vi "Measurements UI_Measure-Scope SP.vi"() -> ()   [LabVIEW 2012]
uses:
  Measurement Operations_Meas.ctl
  Measure Operations_Meas.ctl
  Data Structure.llb/Sub Panel Status Flag_DStr-Scope SP.vi
  SCOPE Acquisition.llb/SCOPE Operations_SA-Scope SP.ctl
  <vilib>/Utility/miscctls.llb/LVStringsAndValuesArrayTypeDef.ctl
panel:
  in  "TempVari":T3={"error"={"status"=FALSE, "code"=0, "source"=""}, "Measure"=refnum, "Message"={"Chans"=[{"String"="0", "Value"=0.0}, {"String"="1", "Value"=1.0}], "LevelRange"={"Max"=10.0, "Min"=-10.0}, "InstruHandle"=""}, "message"=variant, "Item Names"=[], "Config"=[], "InstruHandle"=""}
  in  "Done":bool
  in  "Clear":bool
  in  "Remove":bool
  in  "Add":bool
  in  "List":i32(listbox) caption="标量测量"
  # "操作"
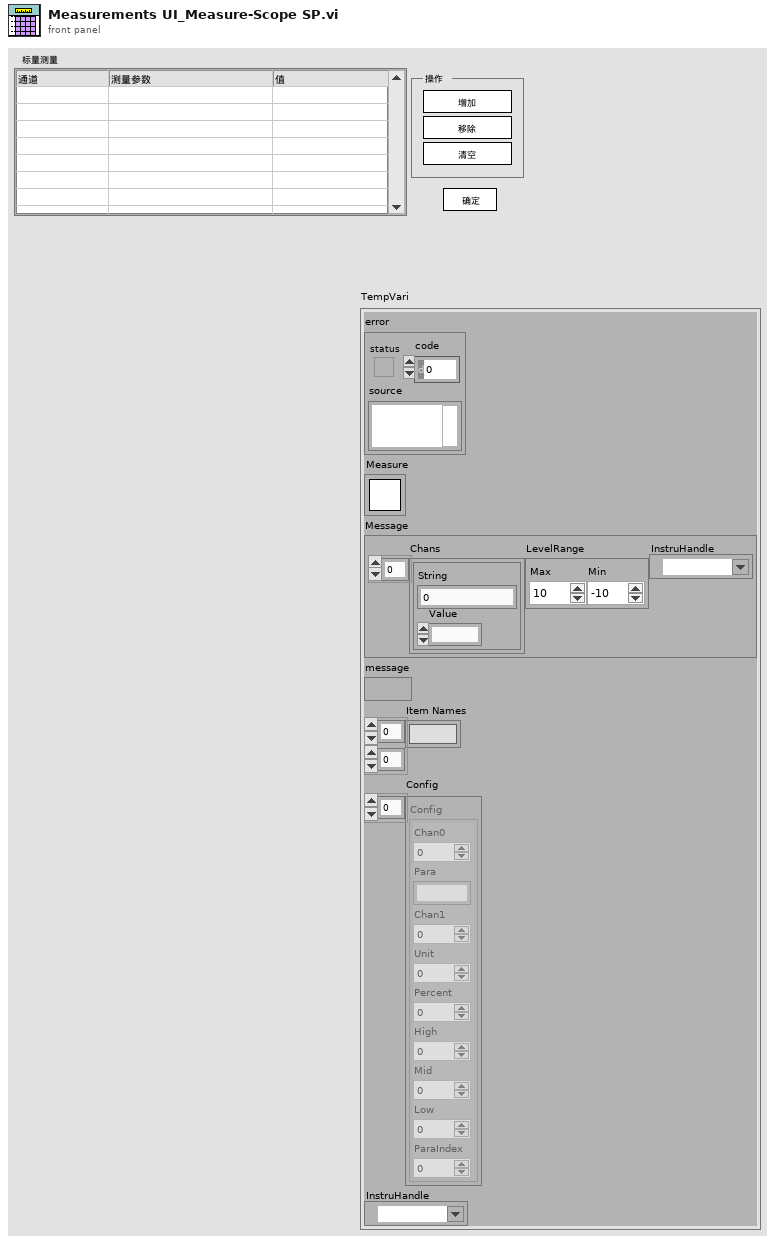
[diagram p1: front panel]
types:
  T1 = typedef "Queue RefNum" = refnum<k1>
  T2 = typedef "LVStringsAndValuesArrayTypeDef.ctl" = cluster{"String":string, "Value":ext}[]
  T3 = cluster{"error":errorcluster, "Measure":T1, "Message":cluster{"Chans":T2, "LevelRange":cluster{"Max":dbl, "Min":dbl}, "InstruHandle":refnum<k15>}, "message":variant, "Item Names":string[][], "Config":cluster{"Chan0":i32, "Para":string, "Chan1":i32, "Unit":i32, "Percent":i32, "High":dbl, "Mid":dbl, "Low":dbl, "ParaIndex":i32}[], "InstruHandle":refnum<k15>}
  T4 = typedef "Measurement Operations_Meas.ctl" = enum16{"Initialize", "Idle", "Add", "Delete", "Clear", "Caculate", "Refresh List Items", "Error Handle", "Close FP", "Exit"}
  T5 = typedef "Measure Operations_Meas.ctl" = enum16{"Add", "Config&Read", "Delete", "Clear"}
  T6 = typedef "SCOPE Operations_SA-Scope SP.ctl" = enum16{"Noop", "Initial", "Horizontal", "Vertical", "Trigger", "RIS", "Initiate", "Fetch", "Abort", "Close", "SelfCalibrate", "AutoSetup"}
  T7 = typedef "Dynamic VI Paths_FS-Scope SP.ctl" = cluster{"Measure":path, "Cursors":path, "Add Para":path, "Config":path}
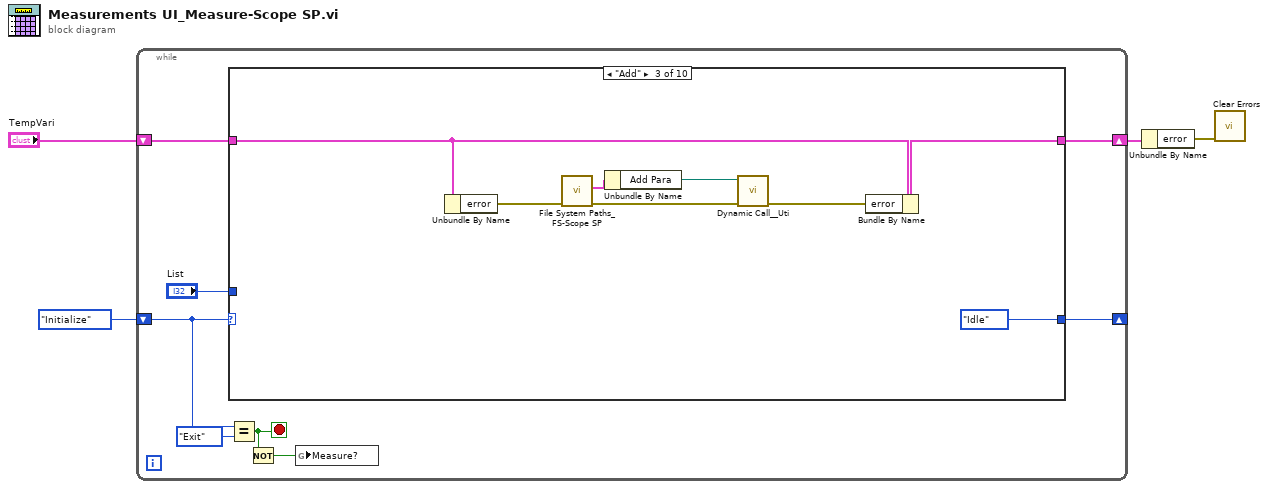
[diagram p0: block diagram]
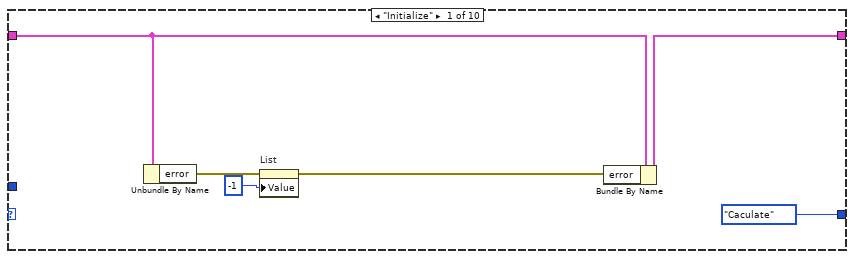
[diagram p2: hidden frame]
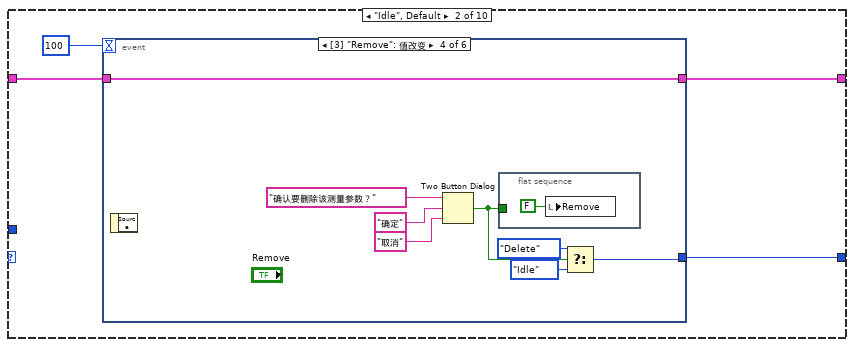
[diagram p3: hidden frame]
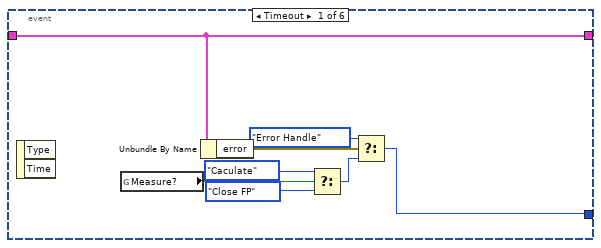
[diagram p4: hidden frame]
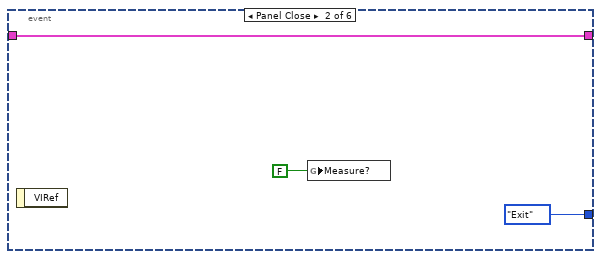
[diagram p5: hidden frame]
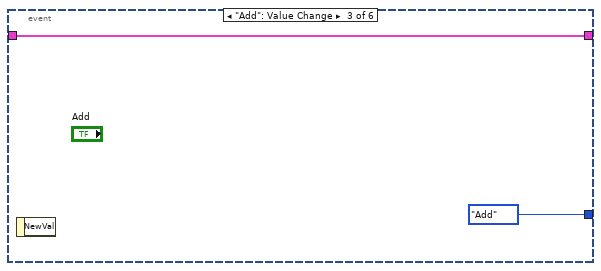
[diagram p6: hidden frame]
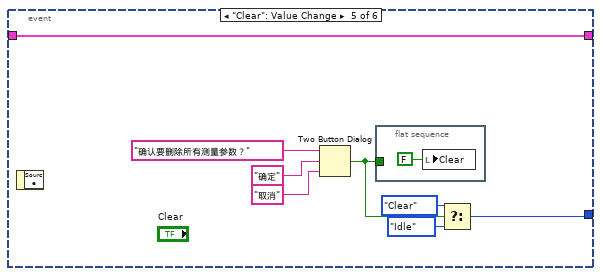
[diagram p7: hidden frame]
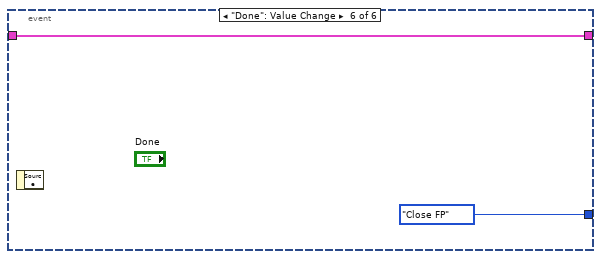
[diagram p8: hidden frame]
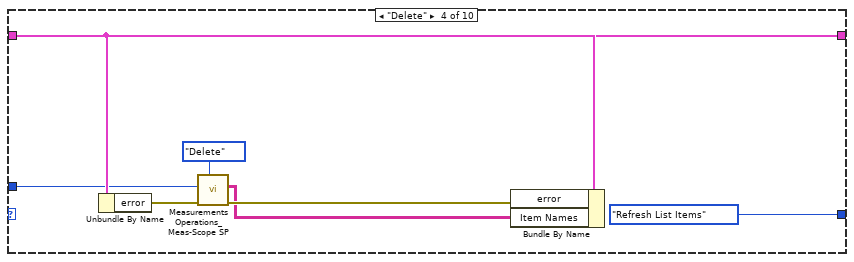
[diagram p9: hidden frame]
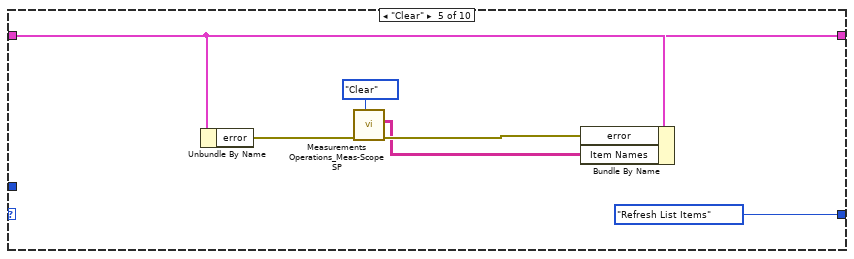
[diagram p10: hidden frame]
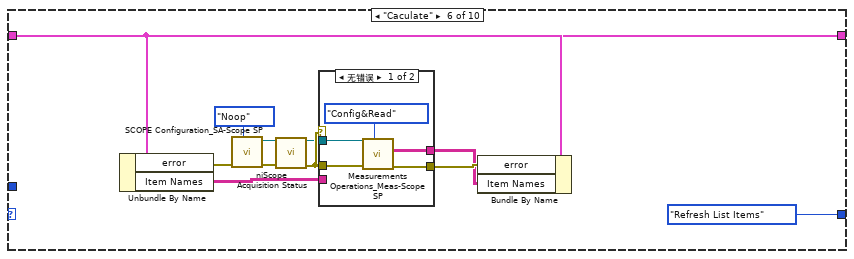
[diagram p11: hidden frame]
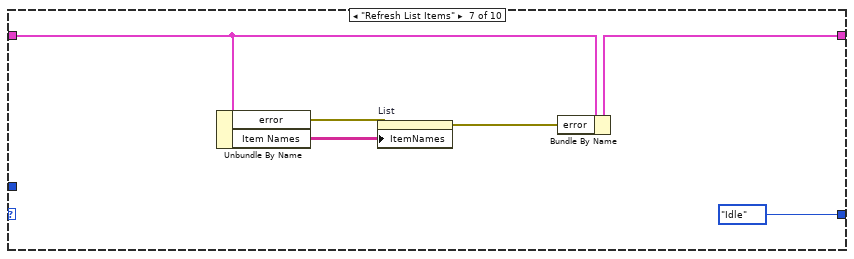
[diagram p13: hidden frame]
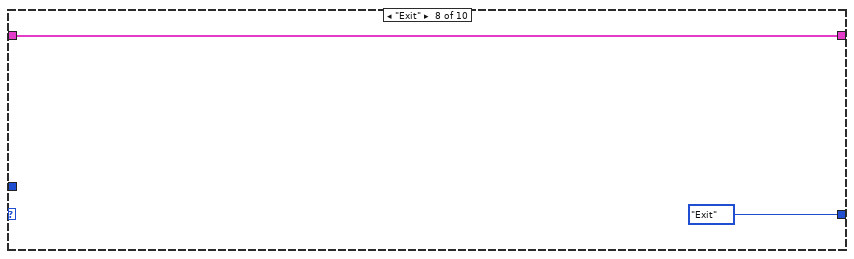
[diagram p14: hidden frame]
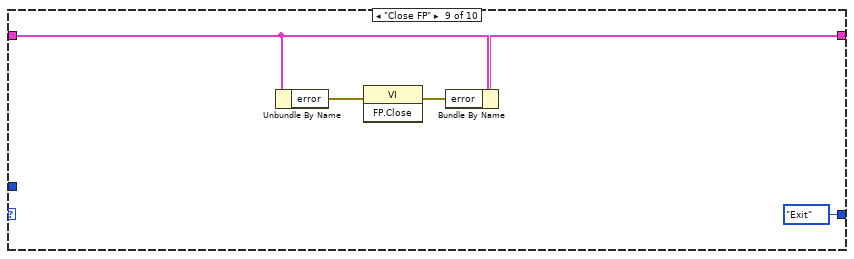
[diagram p15: hidden frame]
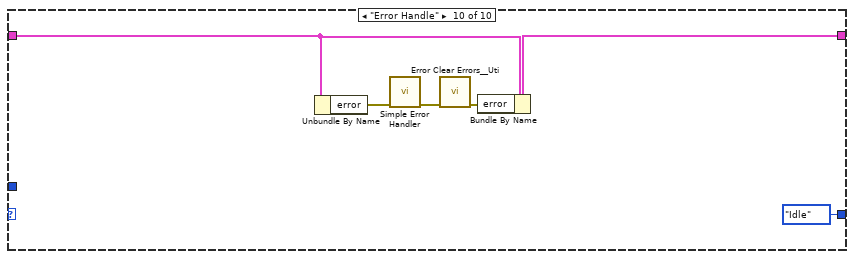
[diagram p16: hidden frame]
diagram:
  n1 = while {
    shift-right: [w12] -> _
    shift-left: Measurement_Operations_Meas."Initialize" ("Operations") -> [w11]
    shift-right: [w7] -> w3
    shift-left: "TempVari" -> [w8]
    stop <- w6 stop-if-true
    n2 = case shown="\"Add\"" w11 {
      tunnel: [Measurement_Operations_Meas."Caculate" ("Operations") w21 Measurement_Operations_Meas."Idle" ("Operations") Measurement_Operations_Meas."Refresh List Items" ("Operations") Measurement_Operations_Meas."Refresh List Items" ("Operations") Measurement_Operations_Meas."Refresh List Items" ("Operations") Measurement_Operations_Meas."Idle" ("Operations") Measurement_Operations_Meas."Exit" ("Operations") Measurement_Operations_Meas."Exit" ("Operations") Measurement_Operations_Meas."Idle" ("Operations")] -> w12
      tunnel: "List" -> [_ _ _ w66 _ _ _ _ _ _]
      tunnel: w8 -> [w16 w20 w60 w70 w77 w88 w99 w103 w108 w113]
      tunnel: [w14 w19 w59 w69 w76 w87 w98 w103 w106 w111] -> w7
      frame "Initialize" {
        n3 = Unbundle By Name(w16) -> ("error"=w15:errorcluster)
        n4 = property on="List" class="MCListbox (严格)"(error in=w15, "Value"=-1 ("List")) -> (error out=w13:errorcluster)  [unwired: 1 in, 1 out]
        n5 = Bundle By Name(cluster=w16, "error"=w13) -> (w14:T3)
      }
      frame "Idle", Default {
        n6 = event shown="[3] \"Remove\": 值改变" {
          selector: _ -> [_ _ _ _ _ _]
          dyn-events: _ -> [_ _ _ _ _ _]
          timeout: 100 -> [_ _ _ _ _ _]
          tunnel: [w23 Measurement_Operations_Meas."Exit" ("Operations") Measurement_Operations_Meas."Add" ("Operations") w37 w46 Measurement_Operations_Meas."Close FP" ("Operations")] -> w21
          tunnel: w20 -> [w27 w33 w34 w36 w45 w54]
          tunnel: [w27 w33 w34 w36 w45 w54] -> w19
          event Timeout {
            n7 = event-data() -> ()  [unwired: 1 in, 2 out]
            n8 = global read "Sub Panel Status Flag_DStr-Scope SP.vi" "Measure?"() -> (w30:bool)
            n9 = Unbundle By Name(w27) -> ("error"=w26:errorcluster)
            n10 = Select(t=Measurement_Operations_Meas."Caculate" ("Operations"), s=w30, f=Measurement_Operations_Meas."Close FP" ("Operations")) -> (s? t:f=w24:T4)
            n11 = Select(t=Measurement_Operations_Meas."Error Handle" ("Operations"), s=w26, f=w24) -> (s? t:f=w23:T4)
          }
          event Panel Close {
            n12 = event-data() -> ()  [unwired: 1 in, 1 out]
            n13 = global write "Sub Panel Status Flag_DStr-Scope SP.vi" "Measure?"(FALSE ("Measure?")) -> ()
          }
          event "Add": Value Change {
            n14 = event-data() -> ()  [unwired: 1 in, 1 out]
          }
          event "Remove": Value Change {
            n15 = event-data() -> ()  [unwired: 1 in, 1 out]
            n16 = Two Button Dialog(message="确认要删除该测量参数？", 1:"取消" ("message"), 2:"确定" ("message")) -> (T button?=w40:bool)
            n17 = flat-sequence {
              tunnel: w40 -> [_]
              frame #0 {
                n18 = local write "Remove"(FALSE ("Clear")) -> ()
              }
            }
            n19 = Select(t=Measurement_Operations_Meas."Delete" ("Operations"), s=w40, f=Measurement_Operations_Meas."Idle" ("Operations")) -> (s? t:f=w37:T4)
          }
          event "Clear": Value Change {
            n20 = event-data() -> ()  [unwired: 1 in, 1 out]
            n21 = Two Button Dialog(message="确认要删除所有测量参数？", 1:"取消" ("message"), 2:"确定" ("message")) -> (T button?=w49:bool)
            n22 = flat-sequence {
              tunnel: w49 -> [_]
              frame #0 {
                n23 = local write "Clear"(FALSE ("Clear")) -> ()
              }
            }
            n24 = Select(t=Measurement_Operations_Meas."Clear" ("Operations"), s=w49, f=Measurement_Operations_Meas."Idle" ("Operations")) -> (s? t:f=w46:T4)
          }
          event "Done": Value Change {
            n25 = event-data() -> ()  [unwired: 1 in, 1 out]
          }
        }
      }
      frame "Add" {
        n26 = Unbundle By Name(w60) -> ("error"=w61:errorcluster)
        n27 = call "File System Paths_FS-Scope SP.vi"("error in"=w61) -> ("error out"=w57:errorcluster, "DynamicVIs"=w62:T7)  [unwired: 8 in, 1 out]
        n28 = Unbundle By Name(w62) -> ("Add Para"=w58:path)
        n29 = call "Dynamic Call__Uti.vi"("error in (no error)"=w57, "vi path"=w58) -> ("error out"=w56:errorcluster)  [unwired: 9 in]
        n30 = Bundle By Name(cluster=w60, "error"=w56) -> (w59:T3)
      }
      frame "Delete" {
        n31 = Unbundle By Name(w70) -> ("error"=w68:errorcluster)
        n32 = call "Measurements Operations_Meas-Scope SP.vi"("Opearte"=Measure_Operations_Meas."Delete", "error in"=w68, "Index"=w66) -> ("error out"=w65:errorcluster, "Items"=w64:string[][])  [unwired: 5 in, 2 out]
        n33 = Bundle By Name(cluster=w70, "error"=w65, "Item Names"=w64) -> (w69:T3)
      }
      frame "Clear" {
        n34 = Unbundle By Name(w77) -> ("error"=w75:errorcluster)
        n35 = call "Measurements Operations_Meas-Scope SP.vi"("Opearte"=Measure_Operations_Meas."Clear", "error in"=w75) -> ("error out"=w73:errorcluster, "Items"=w72:string[][])  [unwired: 6 in, 2 out]
        n36 = Bundle By Name(cluster=w77, "error"=w73, "Item Names"=w72) -> (w76:T3)
      }
      frame "Caculate" {
        n37 = Unbundle By Name(w88) -> ("error"=w82:errorcluster, "Item Names"=w80:string[][])
        n38 = call "SCOPE Configuration_SA-Scope SP.vi"("Operation"=SCOPE_Operations_SA-Scope_SP."Noop", "error in"=w82) -> ("error out"=w83:errorcluster, "InstruHandle"=w84:refnum<k15>)  [unwired: 5 in, 3 out]
        n39 = call <instrlib>:"niScope Acquisition Status.vi"("instrument handle"=w84, "error in"=w83) -> ("instrument handle out"=w79:refnum<k15>, "error out"=w81:errorcluster)  [unwired: 11 in, 1 out]
        n40 = case shown="无错误" w81 {
          tunnel: [w94 _] -> w89
          tunnel: [w93 w96] -> w86
          tunnel: w81 -> [w92 _]
          tunnel: w80 -> [_ w96]
          tunnel: w79 -> [w91 _]
          frame No Error {
            n41 = call "Measurements Operations_Meas-Scope SP.vi"("Opearte"=Measure_Operations_Meas."Config&Read", "error in"=w92, "InstruHandle"=w91) -> ("error out"=w94:errorcluster, "Items"=w93:string[][])  [unwired: 5 in, 2 out]
          }
          frame Error {
          }
        }
        n42 = Bundle By Name(cluster=w88, "error"=w89, "Item Names"=w86) -> (w87:T3)
      }
      frame "Refresh List Items" {
        n43 = Unbundle By Name(w99) -> ("error"=w101:errorcluster, "Item Names"=w102:string[][])
        n44 = property on="List" class="MCListbox (严格)"(error in=w101, "ItemNames"=w102) -> (error out=w100:errorcluster)  [unwired: 1 in, 1 out]
        n45 = Bundle By Name(cluster=w99, "error"=w100) -> (w98:T3)
      }
      frame "Exit" {
      }
      frame "Close FP" {
        n46 = Unbundle By Name(w108) -> ("error"=w109:errorcluster)
        n47 = invoke class="VI" method="FP.Close"(error in=w109) -> (error out=w107:errorcluster)  [unwired: 2 in, 2 out]
        n48 = Bundle By Name(cluster=w108, "error"=w107) -> (w106:T3)
      }
      frame "Error Handle" {
        n49 = Unbundle By Name(w113) -> ("error"=w115:errorcluster)
        n50 = call <vilib>:"Simple Error Handler.vi"("error in (no error)"=w115) -> ("error out"=w114:errorcluster)  [unwired: 4 in, 4 out]
        n51 = call "Error Clear Errors__Uti.vi"("error in (no error)"=w114) -> ("error out"=w112:errorcluster)  [unwired: 6 in]
        n52 = Bundle By Name(cluster=w113, "error"=w112) -> (w111:T3)
      }
    }
    n53 = Equal?(x=w11, y=Measurement_Operations_Meas."Exit") -> (x = y?=w6:bool)
    n54 = Not(x=w6) -> (.not. x?=w5:bool)
    n55 = global write "Sub Panel Status Flag_DStr-Scope SP.vi" "Measure?"(w5) -> ()
  }
  n56 = Unbundle By Name(w3) -> ("error"=w2:errorcluster)
  n57 = call <vilib>:"Clear Errors.vi"("error in (no error)"=w2) -> ()  [unwired: 6 in, 1 out]
